vi "SID4analyzefile.vi"(8 "error in (no error)":errorcluster, 10 "Interferogram path":path, 11 "Refnum in":T2) -> (0 "error out":errorcluster, 1 "Intensity out":sgl[][](array[numeric]), 2 "Image Out":T1, 3 "Refnum out":T2, 5 "Phase out":sgl[][](array[numeric]))   [LabVIEW 2013]
uses:
  Program Files (x86)/SID4_SDK/SDKSID4_Types.llb/Refnum SDKSID4 session.ctl
  <vilib>/vision/Image Controls.llb/IMAQ Image.ctl
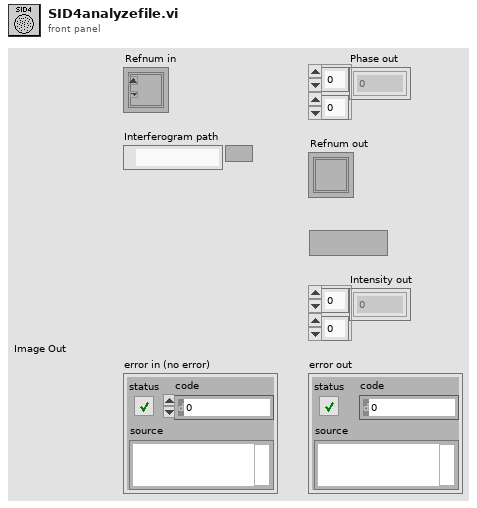
[diagram p1: front panel]
types:
  T1 = typedef "IMAQ Image.ctl" = refnum<image>
  T2 = typedef "Refnum SDKSID4 session.ctl" = refnum<k1>
  T3 = typedef "Image Type" = u32
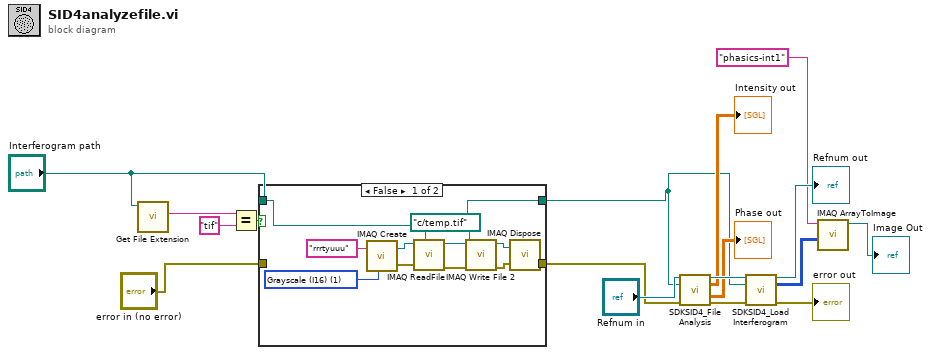
[diagram p0: block diagram]
diagram:
  n1 = call <vilib>:"Get File Extension.vi"("file"="Interferogram path") -> ("lowercase file extension"=w7:string)  [unwired: 7 in, 3 out]
  n2 = Equal?(x=w7, y="tif") -> (x = y?=w5:bool)
  n3 = case shown="False" w5 {
    tunnel: "Interferogram path" -> [w24 w30]
    tunnel: [w18 w30] -> w3
    tunnel: [w19 w29] -> w2
    tunnel: "error in (no error)" -> [_ w29]
    frame False {
      w18 = path "c:/temp.tif" ("File Path")
      w25 = T3 1 items=["Grayscale (U8)", "Grayscale (I16)", "Grayscale (SGL)", "Complex (CSG)", "RGB (U32)", "HSL (U32)", "RGB (U64)", "Grayscale (U16)"] ("Image Type")
      n4 = call "IMAQ Create"("Image Name"="rrrtyuuu", "Image Type"=w25) -> ("New Image"=w27:T1, "error out"=w28:errorcluster)  [unwired: 3 in]
      n5 = call "IMAQ ReadFile"("File Path"=w24, "error in (no error)"=w28, "Image"=w27) -> ("error out"=w20:errorcluster, "Image Out"=w23:T1)  [unwired: 4 in, 3 out]
      n6 = call-poly "IMAQ Write File 2"("error in (no error)"=w20, "File Path"=w18, "Image"=w23) -> ("error out"=w21:errorcluster, "Image Out (duplicate)"=w22:T1)  [unwired: 7 in]
      n7 = call "IMAQ Dispose"("Image"=w22, "error in (no error)"=w21) -> ("error out"=w19:errorcluster)  [unwired: 4 in]
    }
    frame True {
    }
  }
  n8 = call "SDKSID4_File Analysis.vi"("SDKSID4 session In"="Refnum in", "Interferogram File"=w3, "error in (no error)"=w2) -> ("SDKSID4 session Out"=w14:T2, "Intensity out"=→"Intensity out":sgl[][], "Phase out"=→"Phase out":sgl[][], "error out"=w16:errorcluster)  [unwired: 8 in, 1 out]
  n9 = call "SDKSID4_Load Interferogram.vi"("SDKSID4 session In"=w14, "Interferogram File"=w3, "error in (no error)"=w16) -> ("SDKSID4 session Out"=→"Refnum out":T2, "Interferogram[I16]"=w10:i16[][], "error out"=→"error out":errorcluster)  [unwired: 9 in, 1 out]
  n10 = call "IMAQ ArrayToImage"("Image Pixels (I16)"=w10, "Image"="phasics-int1" ("Image Name")) -> ("Image Out"=→"Image Out":T1)  [unwired: 8 in, 1 out]
